vi "Project Dependencies.vi"() -> ()   [LabVIEW 2020, in "GPackScratch.lvlib"]
uses:
  GPackScratch.lvlib
  GPack/PackageAbstract/PackageAbstract.lvclass
panel:
  out "x-y":dbl
  out "error out":errorcluster
  in  "LVProject":path
  in  "Folder":path
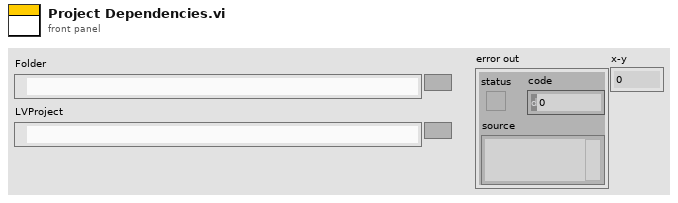
[diagram p1: front panel]
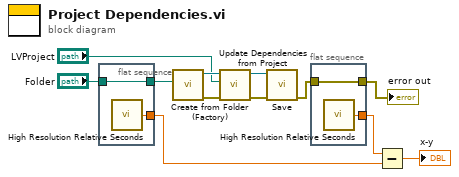
[diagram p0: block diagram]
diagram:
  n1 = flat-sequence {
    tunnel: "Folder" -> [w14]
    tunnel: [w14] -> w6
    tunnel: [w13] -> w2
    frame #0 {
      n2 = call <vilib>:"High Resolution Relative Seconds.vi"() -> ("relative seconds"=w13:dbl)
    }
  }
  n3 = call "Create from Folder (Factory).vi"("Folder"=w6) -> ("error out"=w12:errorcluster, "PackageAbstract out"=w11:refnum<class "PackageAbstract.lvclass">)  [unwired: 9 in]
  n4 = call "Update Dependencies from Project.vi"("error in (no error)"=w12, "lvproj Path"="LVProject", "PackageAbstract in"=w11) -> ("error out"=w9:errorcluster, "PackageAbstract out"=w8:refnum<class "PackageAbstract.lvclass">)  [unwired: 7 in]
  n5 = call "Save.vi"("error in (no error)"=w9, "PackageAbstract in"=w8) -> ("error out"=w5:errorcluster)  [unwired: 8 in, 1 out]
  n6 = flat-sequence {
    tunnel: w5 -> [w16]
    tunnel: [w16] -> w4
    tunnel: [w15] -> w3
    frame #0 {
      n7 = call <vilib>:"High Resolution Relative Seconds.vi"() -> ("relative seconds"=w15:dbl)
    }
  }
  n8 = Subtract(x=w3, y=w2) -> (x-y=→"x-y":dbl)
  "error out" <- w4
